vi "WD_DealData.vi"(2 "mbfDealData":bool, 3 "ArrayIn":u8[](array[numeric]) format="0x%x") -> (0 "ResultArrayOut":string[](array[string]), 1 "mu08BufSize":u8)   [LabVIEW 2011]
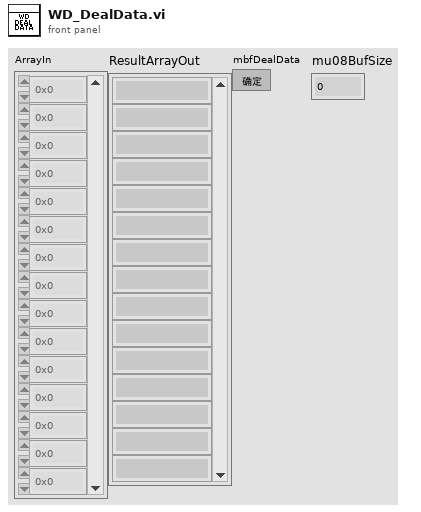
[diagram p1: front panel]
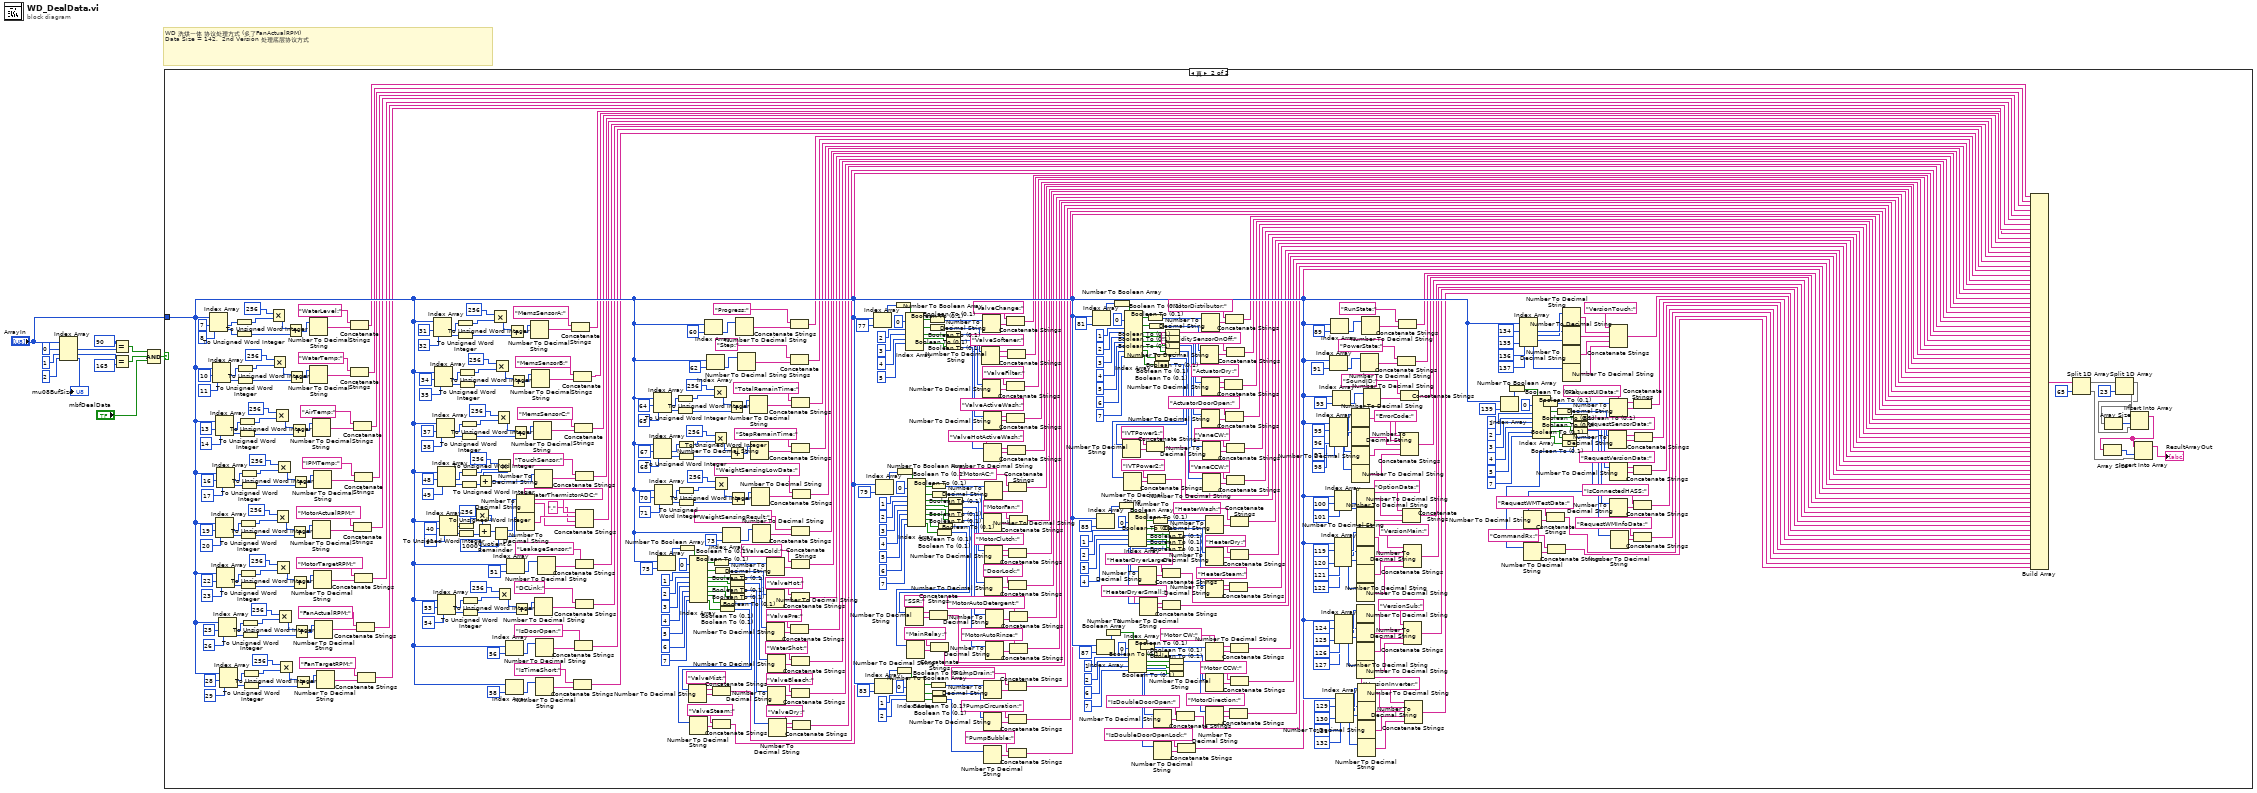
[diagram p0: block diagram]
diagram:
  # "WD 洗烘一体 协议处理方式 (多了FanActualRPM)\nData Size = 142,  2nd Version 处理底层协议方式"
  n1 = Index Array(array="ArrayIn", index #1=0 ("索引"), index #2=1 ("索引"), index #3=2 ("索引")) -> (element #1=w10:u8, element #2=w9:u8, element #3=→"mu08BufSize":u8)
  n2 = Equal?(x=u8 90, y=w10) -> (x = y?=w5:bool)
  n3 = Equal?(x=w9, y=u8 165) -> (x = y?=w4:bool)
  n4 = Compound Arithmetic op=AND(w5, w4, "mbfDealData") -> (w1:bool)
  n5 = case shown="真" w1 {
    tunnel: "ArrayIn" -> [_ w125]
    frame False {
    }
    frame True {
      n6 = Index Array(array=w125, index #1=7 ("索引"), index #2=8 ("索引")) -> (element #1=w673:u8, element #2=w672:u8)
      n7 = Index Array(array=w125, index #1=10 ("索引"), index #2=11 ("索引")) -> (element #1=w659:u8, element #2=w658:u8)
      n8 = Index Array(array=w125, index #1=13 ("索引"), index #2=14 ("索引")) -> (element #1=w649:u8, element #2=w648:u8)
      n9 = Index Array(array=w125, index #1=19 ("索引"), index #2=20 ("索引")) -> (element #1=w626:u8, element #2=w625:u8)
      n10 = Index Array(array=w125, index #1=22 ("索引"), index #2=23 ("索引")) -> (element #1=w615:u8, element #2=w614:u8)
      n11 = Index Array(array=w125, index #1=16 ("索引"), index #2=17 ("索引")) -> (element #1=w637:u8, element #2=w636:u8)
      n12 = Index Array(array=w125, index #1=25 ("索引"), index #2=26 ("索引")) -> (element #1=w604:u8, element #2=w603:u8)
      n13 = Index Array(array=w125, index #1=28 ("索引"), index #2=29 ("索引")) -> (element #1=w593:u8, element #2=w592:u8)
      n14 = To Unsigned Word Integer(number=w673) -> (unsigned 16bit integer=w671:u16)
      n15 = To Unsigned Word Integer(number=w672) -> (unsigned 16bit integer=w668:u16)
      n16 = To Unsigned Word Integer(number=w659) -> (unsigned 16bit integer=w662:u16)
      n17 = To Unsigned Word Integer(number=w658) -> (unsigned 16bit integer=w660:u16)
      n18 = To Unsigned Word Integer(number=w649) -> (unsigned 16bit integer=w652:u16)
      n19 = To Unsigned Word Integer(number=w648) -> (unsigned 16bit integer=w650:u16)
      n20 = To Unsigned Word Integer(number=w626) -> (unsigned 16bit integer=w629:u16)
      n21 = To Unsigned Word Integer(number=w625) -> (unsigned 16bit integer=w627:u16)
      n22 = To Unsigned Word Integer(number=w615) -> (unsigned 16bit integer=w618:u16)
      n23 = To Unsigned Word Integer(number=w614) -> (unsigned 16bit integer=w616:u16)
      n24 = To Unsigned Word Integer(number=w637) -> (unsigned 16bit integer=w640:u16)
      n25 = To Unsigned Word Integer(number=w636) -> (unsigned 16bit integer=w638:u16)
      n26 = To Unsigned Word Integer(number=w604) -> (unsigned 16bit integer=w607:u16)
      n27 = To Unsigned Word Integer(number=w603) -> (unsigned 16bit integer=w605:u16)
      n28 = To Unsigned Word Integer(number=w593) -> (unsigned 16bit integer=w596:u16)
      n29 = To Unsigned Word Integer(number=w592) -> (unsigned 16bit integer=w594:u16)
      n30 = Multiply(x=u16 256, y=w671) -> (x*y=w669:u16)
      n31 = Multiply(x=u16 256, y=w662) -> (x*y=w661:u16)
      n32 = Multiply(x=u16 256, y=w652) -> (x*y=w651:u16)
      n33 = Multiply(x=u16 256, y=w629) -> (x*y=w628:u16)
      n34 = Multiply(x=u16 256, y=w618) -> (x*y=w617:u16)
      n35 = Multiply(x=u16 256, y=w640) -> (x*y=w639:u16)
      n36 = Multiply(x=u16 256, y=w607) -> (x*y=w606:u16)
      n37 = Multiply(x=u16 256, y=w596) -> (x*y=w595:u16)
      n38 = Add(x=w669, y=w668) -> (x+y=w667:u16)
      n39 = Add(x=w661, y=w660) -> (x+y=w655:u16)
      n40 = Add(x=w651, y=w650) -> (x+y=w645:u16)
      n41 = Add(x=w628, y=w627) -> (x+y=w622:u16)
      n42 = Add(x=w617, y=w616) -> (x+y=w611:u16)
      n43 = Add(x=w639, y=w638) -> (x+y=w633:u16)
      n44 = Add(x=w606, y=w605) -> (x+y=w600:u16)
      n45 = Add(x=w595, y=w594) -> (x+y=w589:u16)
      n46 = Number To Decimal String(number=w667) -> (decimal integer string=w666:string)  [unwired: 1 in]
      n47 = Number To Decimal String(number=w655) -> (decimal integer string=w657:string)  [unwired: 1 in]
      n48 = Number To Decimal String(number=w645) -> (decimal integer string=w647:string)  [unwired: 1 in]
      n49 = Number To Decimal String(number=w622) -> (decimal integer string=w624:string)  [unwired: 1 in]
      n50 = Number To Decimal String(number=w611) -> (decimal integer string=w613:string)  [unwired: 1 in]
      n51 = Number To Decimal String(number=w633) -> (decimal integer string=w635:string)  [unwired: 1 in]
      n52 = Number To Decimal String(number=w600) -> (decimal integer string=w602:string)  [unwired: 1 in]
      n53 = Number To Decimal String(number=w589) -> (decimal integer string=w591:string)  [unwired: 1 in]
      n54 = Concatenate Strings("WaterLevel:", w666) -> (w114:string)
      n55 = Concatenate Strings("WaterTemp:", w657) -> (w113:string)
      n56 = Concatenate Strings("AirTemp:", w647) -> (w112:string)
      n57 = Concatenate Strings("MotorActualRPM:", w624) -> (w110:string)
      n58 = Concatenate Strings("MotorTargetRPM:", w613) -> (w109:string)
      n59 = Concatenate Strings("IPMTemp:", w635) -> (w111:string)
      n60 = Concatenate Strings("FanActualRPM:", w602) -> (w108:string)
      n61 = Concatenate Strings("FanTargetRPM:", w591) -> (w107:string)
      n62 = Index Array(array=w125, index #1=31 ("索引"), index #2=32 ("索引")) -> (element #1=w582:u8, element #2=w581:u8)
      n63 = Index Array(array=w125, index #1=34 ("索引"), index #2=35 ("索引")) -> (element #1=w571:u8, element #2=w570:u8)
      n64 = Index Array(array=w125, index #1=37 ("索引"), index #2=38 ("索引")) -> (element #1=w560:u8, element #2=w559:u8)
      n65 = Index Array(array=w125, index #1=48 ("索引"), index #2=49 ("索引")) -> (element #1=w549:u8, element #2=w548:u8)
      n66 = Index Array(array=w125, index #1=53 ("索引"), index #2=54 ("索引")) -> (element #1=w527:u8, element #2=w526:u8)
      n67 = Index Array(array=w125, index #1=40 ("索引"), index #2=41 ("索引")) -> (element #1=w540:u8, element #2=w539:u8)
      n68 = To Unsigned Word Integer(number=w582) -> (unsigned 16bit integer=w585:u16)
      n69 = To Unsigned Word Integer(number=w581) -> (unsigned 16bit integer=w583:u16)
      n70 = To Unsigned Word Integer(number=w540) -> (unsigned 16bit integer=w541:u16)
      n71 = To Unsigned Word Integer(number=w539) -> (unsigned 16bit integer=w32:u16)
      n72 = To Unsigned Word Integer(number=w571) -> (unsigned 16bit integer=w574:u16)
      n73 = To Unsigned Word Integer(number=w570) -> (unsigned 16bit integer=w572:u16)
      n74 = To Unsigned Word Integer(number=w560) -> (unsigned 16bit integer=w563:u16)
      n75 = To Unsigned Word Integer(number=w559) -> (unsigned 16bit integer=w561:u16)
      n76 = To Unsigned Word Integer(number=w549) -> (unsigned 16bit integer=w552:u16)
      n77 = To Unsigned Word Integer(number=w548) -> (unsigned 16bit integer=w550:u16)
      n78 = To Unsigned Word Integer(number=w527) -> (unsigned 16bit integer=w530:u16)
      n79 = To Unsigned Word Integer(number=w526) -> (unsigned 16bit integer=w528:u16)
      n80 = Multiply(x=u16 256, y=w541) -> (x*y=w33:u16)
      n81 = Add(x=w33, y=w32) -> (x+y=w31:u16)
      n82 = Multiply(x=u16 256, y=w585) -> (x*y=w584:u16)
      n83 = Quotient & Remainder(x=w31, y=u16 1000) -> (x-y*floor(x/y)=w29:u16, floor(x/y)=w28:u16)
      n84 = Multiply(x=u16 256, y=w574) -> (x*y=w573:u16)
      n85 = Multiply(x=u16 256, y=w563) -> (x*y=w562:u16)
      n86 = Multiply(x=u16 256, y=w552) -> (x*y=w551:u16)
      n87 = Add(x=w551, y=w550) -> (x+y=w545:u16)
      n88 = Multiply(x=u16 256, y=w530) -> (x*y=w529:u16)
      n89 = Index Array(array=w125, index=56 ("索引")) -> (element=w520:u8)
      n90 = Index Array(array=w125, index=58 ("索引")) -> (element=w516:u8)
      n91 = Index Array(array=w125, index=51 ("索引")) -> (element=w535:u8)
      n92 = Add(x=w584, y=w583) -> (x+y=w578:u16)
      n93 = Add(x=w573, y=w572) -> (x+y=w567:u16)
      n94 = Add(x=w562, y=w561) -> (x+y=w556:u16)
      n95 = Add(x=w529, y=w528) -> (x+y=w523:u16)
      n96 = Number To Decimal String(number=w29) -> (decimal integer string=w26:string)  [unwired: 1 in]
      n97 = Number To Decimal String(number=w28) -> (decimal integer string=w27:string)  [unwired: 1 in]
      n98 = Number To Decimal String(number=w578) -> (decimal integer string=w580:string)  [unwired: 1 in]
      n99 = Number To Decimal String(number=w567) -> (decimal integer string=w569:string)  [unwired: 1 in]
      n100 = Number To Decimal String(number=w556) -> (decimal integer string=w558:string)  [unwired: 1 in]
      n101 = Number To Decimal String(number=w545) -> (decimal integer string=w547:string)  [unwired: 1 in]
      n102 = Number To Decimal String(number=w523) -> (decimal integer string=w525:string)  [unwired: 1 in]
      n103 = Number To Decimal String(number=w520) -> (decimal integer string=w519:string)  [unwired: 1 in]
      n104 = Number To Decimal String(number=w516) -> (decimal integer string=w515:string)  [unwired: 1 in]
      n105 = Number To Decimal String(number=w535) -> (decimal integer string=w534:string)  [unwired: 1 in]
      n106 = Concatenate Strings("MemsSensorA:", w580) -> (w106:string)
      n107 = Concatenate Strings("MemsSensorB:", w569) -> (w105:string)
      n108 = Concatenate Strings("IsTimeShort:", w515) -> (w98:string)
      n109 = Concatenate Strings("IsDoorOpen:", w519) -> (w99:string)
      n110 = Concatenate Strings("MemsSensorC:", w558) -> (w104:string)
      n111 = Concatenate Strings("TouchSensor:", w547) -> (w103:string)
      n112 = Concatenate Strings("LeakageSensor:", w534) -> (w101:string)
      n113 = Concatenate Strings("WaterThermistorADC:", w27, "." ("字符串"), w26) -> (w102:string)
      n114 = Concatenate Strings("DCLink:", w525) -> (w100:string)
      n115 = Index Array(array=w125, index #1=64 ("索引"), index #2=65 ("索引")) -> (element #1=w500:u8, element #2=w499:u8)
      n116 = Index Array(array=w125, index #1=67 ("索引"), index #2=68 ("索引")) -> (element #1=w489:u8, element #2=w488:u8)
      n117 = Index Array(array=w125, index #1=70 ("索引"), index #2=71 ("索引")) -> (element #1=w478:u8, element #2=w477:u8)
      n118 = Index Array(array=w125, index=75 ("索引")) -> (element=w467:u8)
      n119 = To Unsigned Word Integer(number=w500) -> (unsigned 16bit integer=w503:u16)
      n120 = To Unsigned Word Integer(number=w499) -> (unsigned 16bit integer=w501:u16)
      n121 = To Unsigned Word Integer(number=w489) -> (unsigned 16bit integer=w492:u16)
      n122 = To Unsigned Word Integer(number=w488) -> (unsigned 16bit integer=w490:u16)
      n123 = To Unsigned Word Integer(number=w478) -> (unsigned 16bit integer=w481:u16)
      n124 = To Unsigned Word Integer(number=w477) -> (unsigned 16bit integer=w479:u16)
      n125 = Number To Boolean Array(number=w467) -> (Boolean array=w466:bool[])
      n126 = Index Array(array=w466, index #1=0 ("索引"), index #2=1 ("索引"), index #3=2 ("索引"), index #4=3 ("索引"), index #5=4 ("索引"), index #6=5 ("索引"), index #7=6 ("索引"), index #8=7 ("索引")) -> (element #1=w457:bool, element #2=w453:bool, element #3=w447:bool, element #4=w445:bool, element #5=w442:bool, element #6=w437:bool, element #7=w436:bool, element #8=w435:bool)
      n127 = Index Array(array=w125, index=60 ("索引")) -> (element=w513:u8)
      n128 = Index Array(array=w125, index=62 ("索引")) -> (element=w510:u8)
      n129 = Multiply(x=u16 256, y=w503) -> (x*y=w502:u16)
      n130 = Multiply(x=u16 256, y=w492) -> (x*y=w491:u16)
      n131 = Multiply(x=u16 256, y=w481) -> (x*y=w480:u16)
      n132 = Boolean To (0,1)(Boolean=w457) -> (0, 1=w456:i16)
      n133 = Boolean To (0,1)(Boolean=w453) -> (0, 1=w452:i16)
      n134 = Boolean To (0,1)(Boolean=w435) -> (0, 1=w426:i16)
      n135 = Number To Decimal String(number=w426) -> (decimal integer string=w432:string)  [unwired: 1 in]
      n136 = Concatenate Strings("ValveSteam:", w432) -> (w84:string)
      n137 = Boolean To (0,1)(Boolean=w436) -> (0, 1=w427:i16)
      n138 = Number To Decimal String(number=w427) -> (decimal integer string=w434:string)  [unwired: 1 in]
      n139 = Concatenate Strings("ValveMist:", w434) -> (w85:string)
      n140 = Index Array(array=w125, index=73 ("索引")) -> (element=w470:u8)
      n141 = Add(x=w502, y=w501) -> (x+y=w496:u16)
      n142 = Add(x=w491, y=w490) -> (x+y=w485:u16)
      n143 = Boolean To (0,1)(Boolean=w447) -> (0, 1=w446:i16)
      n144 = Boolean To (0,1)(Boolean=w445) -> (0, 1=w443:i16)
      n145 = Boolean To (0,1)(Boolean=w442) -> (0, 1=w438:i16)
      n146 = Boolean To (0,1)(Boolean=w437) -> (0, 1=w428:i16)
      n147 = Add(x=w480, y=w479) -> (x+y=w474:u16)
      n148 = Number To Decimal String(number=w513) -> (decimal integer string=w512:string)  [unwired: 1 in]
      n149 = Number To Decimal String(number=w510) -> (decimal integer string=w509:string)  [unwired: 1 in]
      n150 = Number To Decimal String(number=w496) -> (decimal integer string=w498:string)  [unwired: 1 in]
      n151 = Number To Decimal String(number=w485) -> (decimal integer string=w487:string)  [unwired: 1 in]
      n152 = Number To Decimal String(number=w474) -> (decimal integer string=w476:string)  [unwired: 1 in]
      n153 = Number To Decimal String(number=w470) -> (decimal integer string=w469:string)  [unwired: 1 in]
      n154 = Number To Decimal String(number=w452) -> (decimal integer string=w451:string)  [unwired: 1 in]
      n155 = Number To Decimal String(number=w456) -> (decimal integer string=w455:string)  [unwired: 1 in]
      n156 = Number To Decimal String(number=w446) -> (decimal integer string=w449:string)  [unwired: 1 in]
      n157 = Number To Decimal String(number=w443) -> (decimal integer string=w444:string)  [unwired: 1 in]
      n158 = Number To Decimal String(number=w438) -> (decimal integer string=w441:string)  [unwired: 1 in]
      n159 = Number To Decimal String(number=w428) -> (decimal integer string=w430:string)  [unwired: 1 in]
      n160 = Concatenate Strings("Progress:", w512) -> (w97:string)
      n161 = Concatenate Strings("Step:", w509) -> (w96:string)
      n162 = Concatenate Strings("ValvePre:", w449) -> (w89:string)
      n163 = Concatenate Strings("TotalRemainTime:", w498) -> (w95:string)
      n164 = Concatenate Strings("WeightSensingResult:", w469) -> (w92:string)
      n165 = Concatenate Strings("ValveCold:", w455) -> (w91:string)
      n166 = Concatenate Strings("WaterShot:", w444) -> (w88:string)
      n167 = Concatenate Strings("StepRemainTime:", w487) -> (w94:string)
      n168 = Concatenate Strings("ValveHot:", w451) -> (w90:string)
      n169 = Concatenate Strings("ValveBleach:", w441) -> (w87:string)
      n170 = Concatenate Strings("WeightSensingLowData:", w476) -> (w93:string)
      n171 = Concatenate Strings("ValveDry:", w430) -> (w86:string)
      n172 = Index Array(array=w125, index=77 ("索引")) -> (element=w424:u8)
      n173 = Index Array(array=w125, index=83 ("索引")) -> (element=w297:u8)
      n174 = Index Array(array=w125, index=79 ("索引")) -> (element=w396:u8)
      n175 = Number To Boolean Array(number=w424) -> (Boolean array=w423:bool[])
      n176 = Number To Boolean Array(number=w297) -> (Boolean array=w310:bool[])
      n177 = Number To Boolean Array(number=w396) -> (Boolean array=w395:bool[])
      n178 = Index Array(array=w423, index #1=0 ("索引"), index #2=2 ("索引"), index #3=3 ("索引"), index #4=4 ("索引"), index #5=5 ("索引")) -> (element #1=w417:bool, element #2=w413:bool, element #3=w407:bool, element #4=w405:bool, element #5=w402:bool)  [unwired: 1 in, 1 out]
      n179 = Index Array(array=w310, index #1=0 ("索引"), index #2=1 ("索引"), index #3=2 ("索引")) -> (element #1=w306:bool, element #2=w302:bool, element #3=w298:bool)
      n180 = Index Array(array=w395, index #1=0 ("索引"), index #2=1 ("索引"), index #3=2 ("索引"), index #4=3 ("索引"), index #5=4 ("索引"), index #6=5 ("索引"), index #7=6 ("索引"), index #8=7 ("索引")) -> (element #1=w386:bool, element #2=w382:bool, element #3=w376:bool, element #4=w374:bool, element #5=w371:bool, element #6=w366:bool, element #7=w365:bool, element #8=w364:bool)
      n181 = Boolean To (0,1)(Boolean=w417) -> (0, 1=w416:i16)
      n182 = Boolean To (0,1)(Boolean=w413) -> (0, 1=w412:i16)
      n183 = Boolean To (0,1)(Boolean=w306) -> (0, 1=w305:i16)
      n184 = Boolean To (0,1)(Boolean=w386) -> (0, 1=w385:i16)
      n185 = Boolean To (0,1)(Boolean=w302) -> (0, 1=w301:i16)
      n186 = Boolean To (0,1)(Boolean=w382) -> (0, 1=w381:i16)
      n187 = Boolean To (0,1)(Boolean=w298) -> (0, 1=w295:i16)
      n188 = Boolean To (0,1)(Boolean=w364) -> (0, 1=w355:i16)
      n189 = Number To Decimal String(number=w355) -> (decimal integer string=w361:string)  [unwired: 1 in]
      n190 = Concatenate Strings("MainRelay:", w361) -> (w71:string)
      n191 = Boolean To (0,1)(Boolean=w365) -> (0, 1=w356:i16)
      n192 = Number To Decimal String(number=w356) -> (decimal integer string=w363:string)  [unwired: 1 in]
      n193 = Concatenate Strings("SSR:", w363) -> (w72:string)
      n194 = Boolean To (0,1)(Boolean=w407) -> (0, 1=w406:i16)
      n195 = Boolean To (0,1)(Boolean=w405) -> (0, 1=w403:i16)
      n196 = Boolean To (0,1)(Boolean=w402) -> (0, 1=w398:i16)
      n197 = Boolean To (0,1)(Boolean=w376) -> (0, 1=w375:i16)
      n198 = Boolean To (0,1)(Boolean=w374) -> (0, 1=w372:i16)
      n199 = Boolean To (0,1)(Boolean=w371) -> (0, 1=w367:i16)
      n200 = Boolean To (0,1)(Boolean=w366) -> (0, 1=w357:i16)
      n201 = Number To Decimal String(number=w412) -> (decimal integer string=w411:string)  [unwired: 1 in]
      n202 = Number To Decimal String(number=w416) -> (decimal integer string=w415:string)  [unwired: 1 in]
      n203 = Number To Decimal String(number=w406) -> (decimal integer string=w409:string)  [unwired: 1 in]
      n204 = Number To Decimal String(number=w403) -> (decimal integer string=w404:string)  [unwired: 1 in]
      n205 = Number To Decimal String(number=w301) -> (decimal integer string=w300:string)  [unwired: 1 in]
      n206 = Number To Decimal String(number=w295) -> (decimal integer string=w296:string)  [unwired: 1 in]
      n207 = Number To Decimal String(number=w398) -> (decimal integer string=w401:string)  [unwired: 1 in]
      n208 = Number To Decimal String(number=w381) -> (decimal integer string=w380:string)  [unwired: 1 in]
      n209 = Number To Decimal String(number=w305) -> (decimal integer string=w304:string)  [unwired: 1 in]
      n210 = Number To Decimal String(number=w385) -> (decimal integer string=w384:string)  [unwired: 1 in]
      n211 = Number To Decimal String(number=w375) -> (decimal integer string=w378:string)  [unwired: 1 in]
      n212 = Number To Decimal String(number=w372) -> (decimal integer string=w373:string)  [unwired: 1 in]
      n213 = Number To Decimal String(number=w367) -> (decimal integer string=w370:string)  [unwired: 1 in]
      n214 = Number To Decimal String(number=w357) -> (decimal integer string=w359:string)  [unwired: 1 in]
      n215 = Concatenate Strings("ValveFilter:", w409) -> (w81:string)
      n216 = Concatenate Strings("ValveChange:", w415) -> (w83:string)
      n217 = Concatenate Strings("ValveActiveWash:", w404) -> (w80:string)
      n218 = Concatenate Strings("ValveSoftener:", w411) -> (w82:string)
      n219 = Concatenate Strings("ValveHotActiveWash:", w401) -> (w79:string)
      n220 = Concatenate Strings("MotorClutch:", w378) -> (w76:string)
      n221 = Concatenate Strings("PumpDrain:", w304) -> (w70:string)
      n222 = Concatenate Strings("MotorAC:", w384) -> (w78:string)
      n223 = Concatenate Strings("DoorLock:", w373) -> (w75:string)
      n224 = Concatenate Strings("PumpCircuration:", w300) -> (w69:string)
      n225 = Concatenate Strings("PumpBubble:", w296) -> (w68:string)
      n226 = Concatenate Strings("MotorFan:", w380) -> (w77:string)
      n227 = Concatenate Strings("MotorAutoDetergent:", w370) -> (w74:string)
      n228 = Concatenate Strings("MotorAutoRinse:", w359) -> (w73:string)
      n229 = Index Array(array=w125, index=81 ("索引")) -> (element=w353:u8)
      n230 = Index Array(array=w125, index=85 ("索引")) -> (element=w266:u8)
      n231 = Index Array(array=w125, index=87 ("索引")) -> (element=w264:u8)
      n232 = Number To Boolean Array(number=w264) -> (Boolean array=w263:bool[])
      n233 = Number To Boolean Array(number=w353) -> (Boolean array=w352:bool[])
      n234 = Number To Boolean Array(number=w266) -> (Boolean array=w292:bool[])
      n235 = Index Array(array=w352, index #1=0 ("索引"), index #2=1 ("索引"), index #3=2 ("索引"), index #4=3 ("索引"), index #5=4 ("索引"), index #6=5 ("索引"), index #7=6 ("索引"), index #8=7 ("索引")) -> (element #1=w343:bool, element #2=w339:bool, element #3=w333:bool, element #4=w331:bool, element #5=w328:bool, element #6=w324:bool, element #7=w323:bool, element #8=w322:bool)
      n236 = Index Array(array=w292, index #1=0 ("索引"), index #2=1 ("索引"), index #3=2 ("索引"), index #4=3 ("索引"), index #5=4 ("索引")) -> (element #1=w286:bool, element #2=w282:bool, element #3=w276:bool, element #4=w274:bool, element #5=w271:bool)
      n237 = Index Array(array=w263, index #1=0 ("索引"), index #2=1 ("索引"), index #3=2 ("索引"), index #4=6 ("索引"), index #5=7 ("索引")) -> (element #1=w257:bool, element #2=w253:bool, element #3=w247:bool, element #4=w245:bool, element #5=w242:bool)
      n238 = Boolean To (0,1)(Boolean=w257) -> (0, 1=w256:i16)
      n239 = Boolean To (0,1)(Boolean=w343) -> (0, 1=w342:i16)
      n240 = Boolean To (0,1)(Boolean=w339) -> (0, 1=w338:i16)
      n241 = Boolean To (0,1)(Boolean=w286) -> (0, 1=w285:i16)
      n242 = Boolean To (0,1)(Boolean=w282) -> (0, 1=w281:i16)
      n243 = Boolean To (0,1)(Boolean=w253) -> (0, 1=w252:i16)
      n244 = Boolean To (0,1)(Boolean=w322) -> (0, 1=w314:i16)
      n245 = Number To Decimal String(number=w314) -> (decimal integer string=w319:string)  [unwired: 1 in]
      n246 = Concatenate Strings("IVTPower2:", w319) -> (w60:string)
      n247 = Boolean To (0,1)(Boolean=w323) -> (0, 1=w315:i16)
      n248 = Number To Decimal String(number=w315) -> (decimal integer string=w321:string)  [unwired: 1 in]
      n249 = Concatenate Strings("IVTPower1:", w321) -> (w61:string)
      n250 = Boolean To (0,1)(Boolean=w333) -> (0, 1=w332:i16)
      n251 = Boolean To (0,1)(Boolean=w331) -> (0, 1=w329:i16)
      n252 = Boolean To (0,1)(Boolean=w328) -> (0, 1=w325:i16)
      n253 = Boolean To (0,1)(Boolean=w324) -> (0, 1=w316:i16)
      n254 = Boolean To (0,1)(Boolean=w276) -> (0, 1=w275:i16)
      n255 = Boolean To (0,1)(Boolean=w274) -> (0, 1=w272:i16)
      n256 = Number To Decimal String(number=w272) -> (decimal integer string=w273:string)  [unwired: 1 in]
      n257 = Concatenate Strings("HeaterDryerLarge:", w273) -> (w56:string)
      n258 = Boolean To (0,1)(Boolean=w271) -> (0, 1=w268:i16)
      n259 = Number To Decimal String(number=w268) -> (decimal integer string=w270:string)  [unwired: 1 in]
      n260 = Concatenate Strings("HeaterDryerSmall:", w270) -> (w55:string)
      n261 = Boolean To (0,1)(Boolean=w247) -> (0, 1=w246:i16)
      n262 = Boolean To (0,1)(Boolean=w245) -> (0, 1=w243:i16)
      n263 = Number To Decimal String(number=w243) -> (decimal integer string=w244:string)  [unwired: 1 in]
      n264 = Boolean To (0,1)(Boolean=w242) -> (0, 1=w239:i16)
      n265 = Number To Decimal String(number=w239) -> (decimal integer string=w241:string)  [unwired: 1 in]
      n266 = Concatenate Strings("IsDoubleDoorOpen:", w244) -> (w51:string)
      n267 = Concatenate Strings("IsDoubleDoorOpenLock:", w241) -> (w50:string)
      n268 = Number To Decimal String(number=w338) -> (decimal integer string=w337:string)  [unwired: 1 in]
      n269 = Number To Decimal String(number=w342) -> (decimal integer string=w341:string)  [unwired: 1 in]
      n270 = Number To Decimal String(number=w332) -> (decimal integer string=w335:string)  [unwired: 1 in]
      n271 = Number To Decimal String(number=w329) -> (decimal integer string=w330:string)  [unwired: 1 in]
      n272 = Number To Decimal String(number=w325) -> (decimal integer string=w327:string)  [unwired: 1 in]
      n273 = Number To Decimal String(number=w316) -> (decimal integer string=w317:string)  [unwired: 1 in]
      n274 = Number To Decimal String(number=w281) -> (decimal integer string=w280:string)  [unwired: 1 in]
      n275 = Number To Decimal String(number=w252) -> (decimal integer string=w251:string)  [unwired: 1 in]
      n276 = Number To Decimal String(number=w285) -> (decimal integer string=w284:string)  [unwired: 1 in]
      n277 = Number To Decimal String(number=w275) -> (decimal integer string=w278:string)  [unwired: 1 in]
      n278 = Number To Decimal String(number=w256) -> (decimal integer string=w255:string)  [unwired: 1 in]
      n279 = Number To Decimal String(number=w246) -> (decimal integer string=w249:string)  [unwired: 1 in]
      n280 = Concatenate Strings("ActuatorDry:", w335) -> (w65:string)
      n281 = Concatenate Strings("MotorDistributor:", w341) -> (w67:string)
      n282 = Concatenate Strings("ActuatorDoorOpen:", w330) -> (w64:string)
      n283 = Concatenate Strings("TurbiditySensorOnOff:", w337) -> (w66:string)
      n284 = Concatenate Strings("VaneCW:", w327) -> (w63:string)
      n285 = Concatenate Strings("VaneCCW:", w317) -> (w62:string)
      n286 = Concatenate Strings("HeaterSteam:", w278) -> (w57:string)
      n287 = Concatenate Strings("MotorDirection:", w249) -> (w52:string)
      n288 = Concatenate Strings("HeaterWash:", w284) -> (w59:string)
      n289 = Concatenate Strings("Motor CW:", w255) -> (w54:string)
      n290 = Concatenate Strings("HeaterDry:", w280) -> (w58:string)
      n291 = Concatenate Strings("Motor CCW:", w251) -> (w53:string)
      n292 = Index Array(array=w125, index=91 ("索引")) -> (element=w232:u8)
      n293 = Index Array(array=w125, index #1=95 ("索引"), index #2=96 ("索引"), index #3=97 ("索引"), index #4=98 ("索引")) -> (element #1=w221:u8, element #2=w220:u8, element #3=w219:u8, element #4=w218:u8)
      n294 = Index Array(array=w125, index=89 ("索引")) -> (element=w236:u8)
      n295 = Index Array(array=w125, index=93 ("索引")) -> (element=w228:u8)
      n296 = Index Array(array=w125, index #1=100 ("索引"), index #2=101 ("索引")) -> (element #1=w211:u8, element #2=w210:u8)
      n297 = Index Array(array=w125, index #1=119 ("索引"), index #2=120 ("索引"), index #3=121 ("索引"), index #4=122 ("索引")) -> (element #1=w201:u8, element #2=w200:u8, element #3=w199:u8, element #4=w198:u8)
      n298 = Index Array(array=w125, index #1=124 ("索引"), index #2=125 ("索引"), index #3=126 ("索引"), index #4=127 ("索引")) -> (element #1=w188:u8, element #2=w187:u8, element #3=w186:u8, element #4=w185:u8)
      n299 = Index Array(array=w125, index #1=129 ("索引"), index #2=130 ("索引"), index #3=131 ("索引"), index #4=132 ("索引")) -> (element #1=w175:u8, element #2=w174:u8, element #3=w173:u8, element #4=w172:u8)
      n300 = Number To Decimal String(number=w221) -> (decimal integer string=w216:string)  [unwired: 1 in]
      n301 = Number To Decimal String(number=w220) -> (decimal integer string=w215:string)  [unwired: 1 in]
      n302 = Number To Decimal String(number=w219) -> (decimal integer string=w214:string)  [unwired: 1 in]
      n303 = Number To Decimal String(number=w218) -> (decimal integer string=w213:string)  [unwired: 1 in]
      n304 = Number To Decimal String(number=w201) -> (decimal integer string=w197:string)  [unwired: 1 in]
      n305 = Number To Decimal String(number=w200) -> (decimal integer string=w196:string)  [unwired: 1 in]
      n306 = Number To Decimal String(number=w199) -> (decimal integer string=w194:string)  [unwired: 1 in]
      n307 = Number To Decimal String(number=w198) -> (decimal integer string=w193:string)  [unwired: 1 in]
      n308 = Number To Decimal String(number=w211) -> (decimal integer string=w208:string)  [unwired: 1 in]
      n309 = Number To Decimal String(number=w210) -> (decimal integer string=w207:string)  [unwired: 1 in]
      n310 = Number To Decimal String(number=w188) -> (decimal integer string=w184:string)  [unwired: 1 in]
      n311 = Number To Decimal String(number=w187) -> (decimal integer string=w183:string)  [unwired: 1 in]
      n312 = Number To Decimal String(number=w186) -> (decimal integer string=w182:string)  [unwired: 1 in]
      n313 = Number To Decimal String(number=w185) -> (decimal integer string=w181:string)  [unwired: 1 in]
      n314 = Number To Decimal String(number=w175) -> (decimal integer string=w171:string)  [unwired: 1 in]
      n315 = Number To Decimal String(number=w174) -> (decimal integer string=w170:string)  [unwired: 1 in]
      n316 = Number To Decimal String(number=w173) -> (decimal integer string=w169:string)  [unwired: 1 in]
      n317 = Number To Decimal String(number=w172) -> (decimal integer string=w168:string)  [unwired: 1 in]
      n318 = Number To Decimal String(number=w232) -> (decimal integer string=w231:string)  [unwired: 1 in]
      n319 = Number To Decimal String(number=w236) -> (decimal integer string=w235:string)  [unwired: 1 in]
      n320 = Number To Decimal String(number=w228) -> (decimal integer string=w227:string)  [unwired: 1 in]
      n321 = Concatenate Strings("PowerState:", w231) -> (w48:string)
      n322 = Concatenate Strings("RunState:", w235) -> (w49:string)
      n323 = Concatenate Strings("SoundID:", w227) -> (w47:string)
      n324 = Concatenate Strings("ErrorCode:", w216, w215, w214, w213) -> (w46:string)
      n325 = Concatenate Strings("OptionData:", w208, w207) -> (w45:string)
      n326 = Concatenate Strings("VersionMain:", w197, w196, w194, w193) -> (w44:string)
      n327 = Concatenate Strings("VersionSub:", w184, w183, w182, w181) -> (w43:string)
      n328 = Concatenate Strings("VersionInverter:", w171, w170, w169, w168) -> (w42:string)
      n329 = Index Array(array=w125, index=139 ("索引")) -> (element=w152:u8)
      n330 = Number To Boolean Array(number=w152) -> (Boolean array=w151:bool[])
      n331 = Index Array(array=w125, index #1=134 ("索引"), index #2=135 ("索引"), index #3=136 ("索引"), index #4=137 ("索引")) -> (element #1=w162:u8, element #2=w161:u8, element #3=w160:u8, element #4=w159:u8)
      n332 = Index Array(array=w151, index #1=0 ("索引"), index #2=1 ("索引"), index #3=2 ("索引"), index #4=3 ("索引"), index #5=4 ("索引"), index #6=5 ("索引"), index #7=7 ("索引")) -> (element #1=w145:bool, element #2=w141:bool, element #3=w135:bool, element #4=w133:bool, element #5=w130:bool, element #6=w122:bool, element #7=w121:bool)
      n333 = Boolean To (0,1)(Boolean=w145) -> (0, 1=w144:i16)
      n334 = Boolean To (0,1)(Boolean=w141) -> (0, 1=w140:i16)
      n335 = Boolean To (0,1)(Boolean=w122) -> (0, 1=w116:i16)
      n336 = Number To Decimal String(number=w116) -> (decimal integer string=w120:string)  [unwired: 1 in]
      n337 = Concatenate Strings("RequestWMTestData:", w120) -> (w35:string)
      n338 = Boolean To (0,1)(Boolean=w121) -> (0, 1=w115:i16)
      n339 = Number To Decimal String(number=w115) -> (decimal integer string=w119:string)  [unwired: 1 in]
      n340 = Concatenate Strings("CommandRx:", w119) -> (w34:string)
      n341 = Number To Decimal String(number=w162) -> (decimal integer string=w158:string)  [unwired: 1 in]
      n342 = Number To Decimal String(number=w161) -> (decimal integer string=w157:string)  [unwired: 1 in]
      n343 = Number To Decimal String(number=w160) -> (decimal integer string=w156:string)  [unwired: 1 in]
      n344 = Number To Decimal String(number=w159) -> (decimal integer string=w155:string)  [unwired: 1 in]
      n345 = Boolean To (0,1)(Boolean=w135) -> (0, 1=w134:i16)
      n346 = Boolean To (0,1)(Boolean=w133) -> (0, 1=w131:i16)
      n347 = Boolean To (0,1)(Boolean=w130) -> (0, 1=w127:i16)
      n348 = Number To Decimal String(number=w140) -> (decimal integer string=w139:string)  [unwired: 1 in]
      n349 = Concatenate Strings("VersionTouch:", w158, w157, w156, w155) -> (w41:string)
      n350 = Number To Decimal String(number=w144) -> (decimal integer string=w143:string)  [unwired: 1 in]
      n351 = Number To Decimal String(number=w134) -> (decimal integer string=w137:string)  [unwired: 1 in]
      n352 = Number To Decimal String(number=w131) -> (decimal integer string=w132:string)  [unwired: 1 in]
      n353 = Number To Decimal String(number=w127) -> (decimal integer string=w129:string)  [unwired: 1 in]
      n354 = Concatenate Strings("RequestVersionData:", w137) -> (w38:string)
      n355 = Concatenate Strings("IsConnectedHASS:", w132) -> (w37:string)
      n356 = Concatenate Strings("RequestUIData:", w143) -> (w40:string)
      n357 = Concatenate Strings("RequestWMInfoData:", w129) -> (w36:string)
      n358 = Concatenate Strings("RequestSensorData:", w139) -> (w39:string)
      n359 = Build Array(w114, w113, w112, w111, w110, w109, w108, w107, w106, w105, w104, w103, w102, w101, w100, w99, w98, w97, w96, w95, w94, w93, w92, w91, w90, w89, w88, w87, w86, w85, w84, w83, w82, w81, w80, w79, w78, w77, w76, w75, w74, w73, w72, w71, w70, w69, w68, w67, w66, w65, w64, w63, w62, w61, w60, w59, w58, w57, w56, w55, w54, w53, w52, w51, w50, w49, w48, w47, w46, w45, w44, w43, w42, w41, w40, w39, w38, w37, w36, w35, w34) -> (w23:string[])
      n360 = Split 1D Array(array=w23, index=65 ("索引")) -> (first subarray=w22:string[], second subarray=w15:string[])
      n361 = Split 1D Array(array=w22, index=23 ("索引")) -> (first subarray=w18:string[], second subarray=w20:string[])
      n362 = Array Size(array=w20) -> (size(s)=w19:i32)
      n363 = Insert Into Array(array=w20, index=w19, new element=w18) -> (w17:string[])
      n364 = Array Size(array=w17) -> (size(s)=w16:i32)
      n365 = Insert Into Array(array=w17, index=w16, new element=w15) -> (→"ResultArrayOut":string[])
    }
  }
